vi "Logrecorder.vi"(1 "error in":errorcluster, 3 "Msg":string) -> (0 "error out":errorcluster)   [LabVIEW 2011]
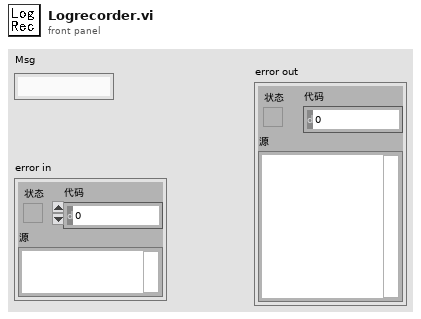
[diagram p1: front panel]
types:
  T1 = enum16{"open", "replace", "create", "open or create", "replace or create", "replace or create with confirmation"}
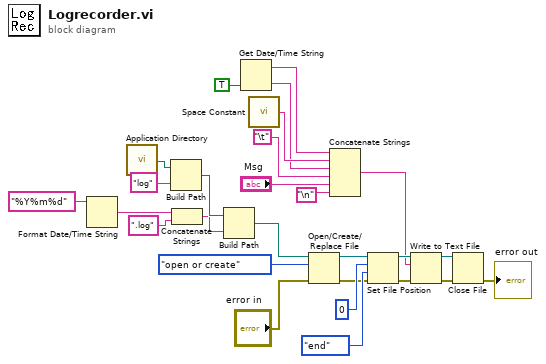
[diagram p0: block diagram]
diagram:
  n1 = Format Date/Time String(time format string (%c)="%Y%m%d" ("时间格式字符串(%c)")) -> (date/time string=w5:string)  [unwired: 2 in]
  n2 = call <vilib>:"Application Directory.vi"() -> ("Application Directory"=w8:path)
  n3 = Build Path(base path=w8, name or relative path="log" ("名称或相对路径")) -> (appended path=w3:path)
  n4 = Concatenate Strings(w5, ".log" ("字符串")) -> (w2:string)
  n5 = Build Path(base path=w3, name or relative path=w2) -> (appended path=w1:path)
  n6 = Get Date/Time String(want seconds? (F)=TRUE ("需要秒？(F)")) -> (date string=w23:string, time string=w21:string)  [unwired: 2 in]
  n7 = call <vilib>:"Space Constant.vi"() -> ("String"=w22:string)
  n8 = Open/Create/Replace File(file path (use dialog)=w1, error in="error in", operation (0:open)=T1."open or create" ("操作(0:open)")) -> (refnum out=w27:refnum<file>, error out=w16:errorcluster)  [unwired: 3 in, 1 out]
  n9 = Concatenate Strings(w23, w22, w21, "\t", "Msg", "\n") -> (w18:string)
  n10 = Set File Position(offset (in bytes) (0)=i64 0 ("偏移量（字节）（0）"), refnum=w27, from (0:start)=enum16{"start", "end", "current"}."end" ("自（0:起始）"), error in=w16) -> (refnum out=w25:refnum<file>, error out=w15:errorcluster)
  n11 = Write to Text File(file (use dialog)=w25, text=w18, error in=w15) -> (refnum out=w13:refnum<file>, error out=w12:errorcluster)  [unwired: 1 in, 1 out]
  n12 = Close File(refnum=w13, error in=w12) -> (error out=→"error out":errorcluster)  [unwired: 1 out]
